vi "FTW-Actor-Initialized.vi"(0 "FTW Actor Instance":refnum<class "FTW-TestStep-Base.lvclass">, 5 "Initialized Response":string, 9 "Positive Init?":string, 11 "error in":errorcluster) -> (4 "FTW Actor Instance out":refnum<class "FTW-TestStep-Base.lvclass">, 15 "error out":errorcluster)   [LabVIEW 2015, in "FTW-TestStep-Base.lvclass"]
uses:
  FTW-TestStep-Base.lvclass
  source/JSON/FTW-JSON-JoinMode.ctl
  FTW-TestStep-Base.lvclass/FTW-TestStep-Base.ctl
  source/actor/Instance-Extended/FTW-ActorExtended.lvclass
panel:
  # "Inputs"
  # "Outputs"
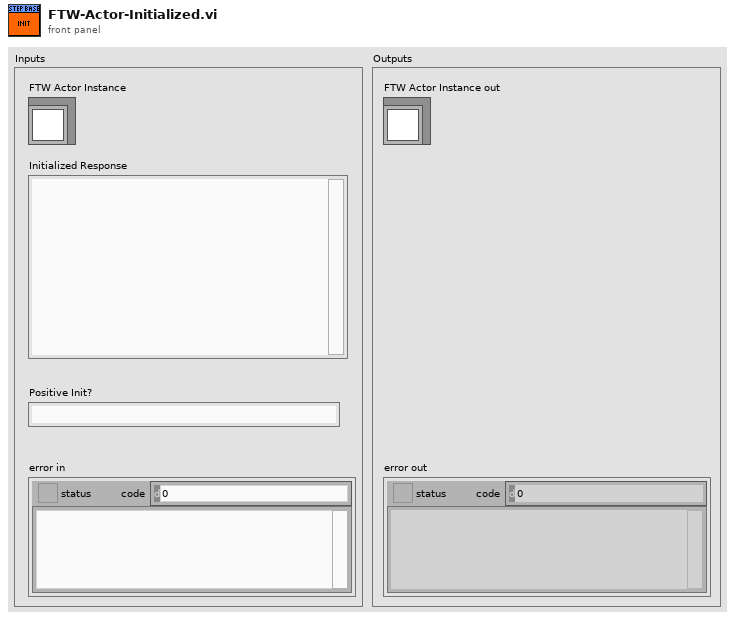
[diagram p1: front panel]
types:
  T1 = typedef "FTW-JSON-JoinMode.ctl" = enum32{"Upsert", "Update Only", "Insert Only"}
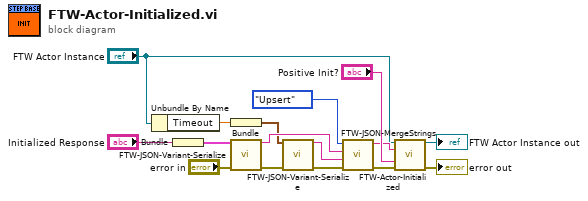
[diagram p0: block diagram]
diagram:
  n1 = Unbundle By Name("FTW Actor Instance") -> ("Timeout"=w1:dbl)
  n2 = Bundle("Initialized Response"="Initialized Response") -> (w10:cluster{"Initialized Response":string})  [unwired: 1 in]
  n3 = Bundle("Timeout"=w1) -> (w2:cluster{"Timeout":dbl})  [unwired: 1 in]
  n4 = call "FTW-JSON-Variant-Serialize.vi"("Variant"=w10, "error in"="error in") -> ("JSON String"=w8:string, "error out"=w11:errorcluster)  [unwired: 12 in]
  n5 = call "FTW-JSON-Variant-Serialize.vi"("Variant"=w2, "error in"=w11) -> ("JSON String"=w5:string, "error out"=w6:errorcluster)  [unwired: 12 in]
  n6 = call "FTW-JSON-MergeStrings.vi"("error in (no error)"=w6, "Initial JSON String (\"\")"=w5, "JSON string to merge (\"\")"=w8, "Update Mode (0: Upsert)"=FTW-JSON-JoinMode."Upsert") -> ("error out"=w9:errorcluster, "Merged JSON String (UTF-8)"=w7:string)  [unwired: 6 in]
  n7 = call-parent "FTW-Actor-Initialized.vi"("FTW Actor Instance"="FTW Actor Instance", "Initialized Response"=w7, "Positive Init?"="Positive Init?", "error in"=w9) -> ("FTW Actor Instance out"=→"FTW Actor Instance out":refnum<class "FTW-TestStep-Base.lvclass">, "error out"=→"error out":errorcluster)  [unwired: 10 in]
